vi "Append New Page.vi"(0 "PDF Report":refnum<class "PDF Report Class.lvclass">, 11 "error in (no error)":errorcluster) -> (4 "PDF Report duplicate":refnum<class "PDF Report Class.lvclass">, 15 "error OUT":errorcluster)   [LabVIEW 2019]
doc: "Creates a page break within the PDF report. \n\nBlank page: iTextSharp won't create the page until you put something on it (like a line feed).\n\n<B>FRANÇAIS</B>\nAjoute un saut de page au rapport PDF.\n\nPage vierge: iTextSharp ne va pas créer une page vide à moins que vous écrivez quelque chose (par exemple un Line Feed).\n\nVersion 1.0\nDeveloped by Jean-Marc Simard\nCopyright © 2010, Exaprom Inc.\nAll rights reserved.\nLicense: BSD\n\nWith iTextSharp 4.1.6 (http://itextsharp.sourceforge.net)\nunder Mozilla Public License Version 1.1\n(http://www.mozilla.org/MPL/MPL-1.1.html)"
uses:
  <userlib>/Exaprom PDF/LV Class/PDF Report Class/PDF Report Class.lvclass
  C:/Program Files/National Instruments/LabVIEW 2019/user.lib/Exaprom PDF/DLL/itextsharp.dll
  DLL/itextsharp.dll
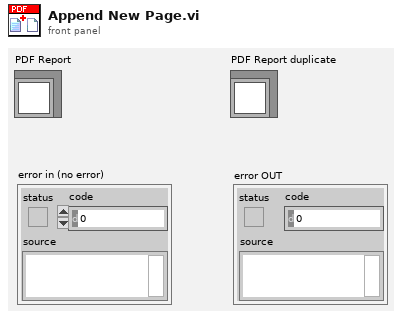
[diagram p1: front panel]
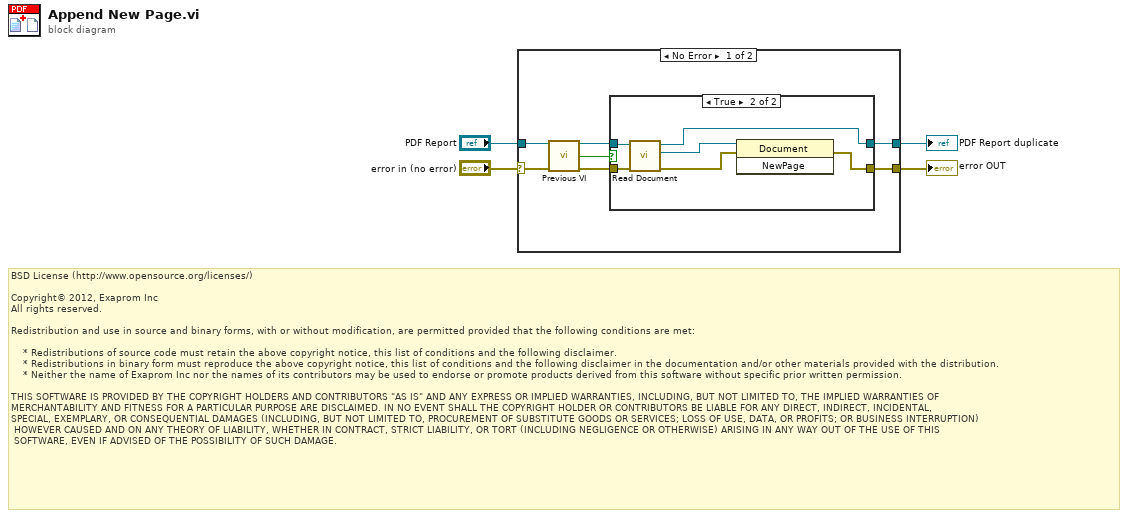
[diagram p0: block diagram]
diagram:
  # "BSD License (http://www.opensource.org/licenses/)\n\nCopyright© 2012, Exaprom Inc\nAll rights reserved.\n\nRedistribution and use in source and binary forms, with or without modification, are permitted provided that the following conditions are met:\n\n    * Redistributions of source code must retain the above copyright notice, this list of conditions and the following disclaimer.\n    * Redistributions in binary form must reproduce the above copyright notice, this list of conditions and the following disclaimer in the documentation and/or other materials provided with the distribution.\n    * Neither the name of Exaprom Inc nor the names of its contributors may be used to endorse or promote products derived from this software without specific prior written permission.\n\nTHIS SOFTWARE IS PROVIDED BY THE COPYRIGHT HOLDERS AND CONTRIBUTORS \"AS IS\" AND ANY EXPRESS OR IMPLIED WARRANTIES, INCLUDING, BUT NOT LIMITED TO, THE IMPLIED WARRANTIES OF \nMERCHANTABILITY AND FITNESS FOR A PARTICULAR PURPOSE ARE DISCLAIMED. IN NO EVENT SHALL THE COPYRIGHT HOLDER OR CONTRIBUTORS BE LIABLE FOR ANY DIRECT, INDIRECT, INCIDENTAL,\nSPECIAL, EXEMPLARY, OR CONSEQUENTIAL DAMAGES (INCLUDING, BUT NOT LIMITED TO, PROCUREMENT OF SUBSTITUTE GOODS OR SERVICES; LOSS OF USE, DATA, OR PROFITS; OR BUSINESS INTERRUPTION)\n HOWEVER CAUSED AND ON ANY THEORY OF LIABILITY, WHETHER IN CONTRACT, STRICT LIABILITY, OR TORT (INCLUDING NEGLIGENCE OR OTHERWISE) ARISING IN ANY WAY OUT OF THE USE OF THIS\n SOFTWARE, EVEN IF ADVISED OF THE POSSIBILITY OF SUCH DAMAGE."
  n1 = case shown="No Error" "error in (no error)" {
    selector: "error in (no error)" -> [w6 w21]
    tunnel: [w9 w21] -> w4
    tunnel: [w10 w20] -> w2
    tunnel: "PDF Report" -> [w11 w20]
    frame No Error {
      n2 = call <userlib>:"Previous VI.vi"("PDF Report IN"=w11, "error in (no error)"=w6) -> ("PDF Report OUT"=w8:refnum<class "PDF Report Class.lvclass">, "Execute Actual VI"=w7:bool, "error out"=w5:errorcluster)  [unwired: 11 out]
      n3 = case shown="True" w7 {
        tunnel: [w13 w15] -> w10
        tunnel: [w12 w19] -> w9
        tunnel: w8 -> [w13 w16]
        tunnel: w5 -> [w12 w18]
        frame False {
        }
        frame True {
          n4 = call-dynamic "Read Document.vi"("error in (no error)"=w18, "PDF Report Class in"=w16) -> ("error out"=w17:errorcluster, "Document"=w14:refnum<k24>, "PDF Report Class out"=w15:refnum<class "PDF Report Class.lvclass">)  [unwired: 7 in]
          n5 = invoke class="Document" method="NewPage"(reference=w14, error in=w17) -> (error out=w19:errorcluster)  [unwired: 1 in, 2 out]
        }
      }
    }
    frame Error {
    }
  }
  "error OUT" <- w4
  "PDF Report duplicate" <- w2
